vi "GVSGet Window Temp Reference.vi"(8 "sWindowName":string, 9 "sVIFullName":path, 10 "pVIRef_In":refnum<vi>, 11 "sAction":string) -> (0 "bResult":bool=TRUE, 1 "nWinType":i32, 2 "sTitleName Out":string, 3 "pVIRef_Out":refnum<vi>, 4 "sIcon_Out":string)   [LabVIEW 2013]
uses:
  <vilib>/Utility/miscctls.llb/LVPointTypeDef.ctl
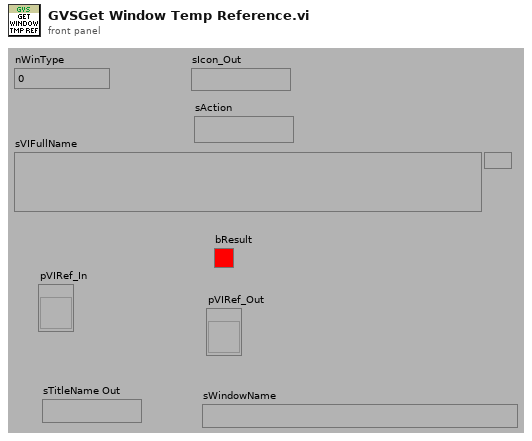
[diagram p1: front panel]
types:
  T1 = enum32{"Invalid", "Default", "Floating", "Floating/Auto-Hide", "Modal"}
  T2 = enum32{"Invalid", "Standard", "Closed", "Hidden", "Minimized", "Maximized"}
  T3 = typedef "LVPointTypeDef.ctl" = cluster{"Horizontal":i16, "Vertical":i16}
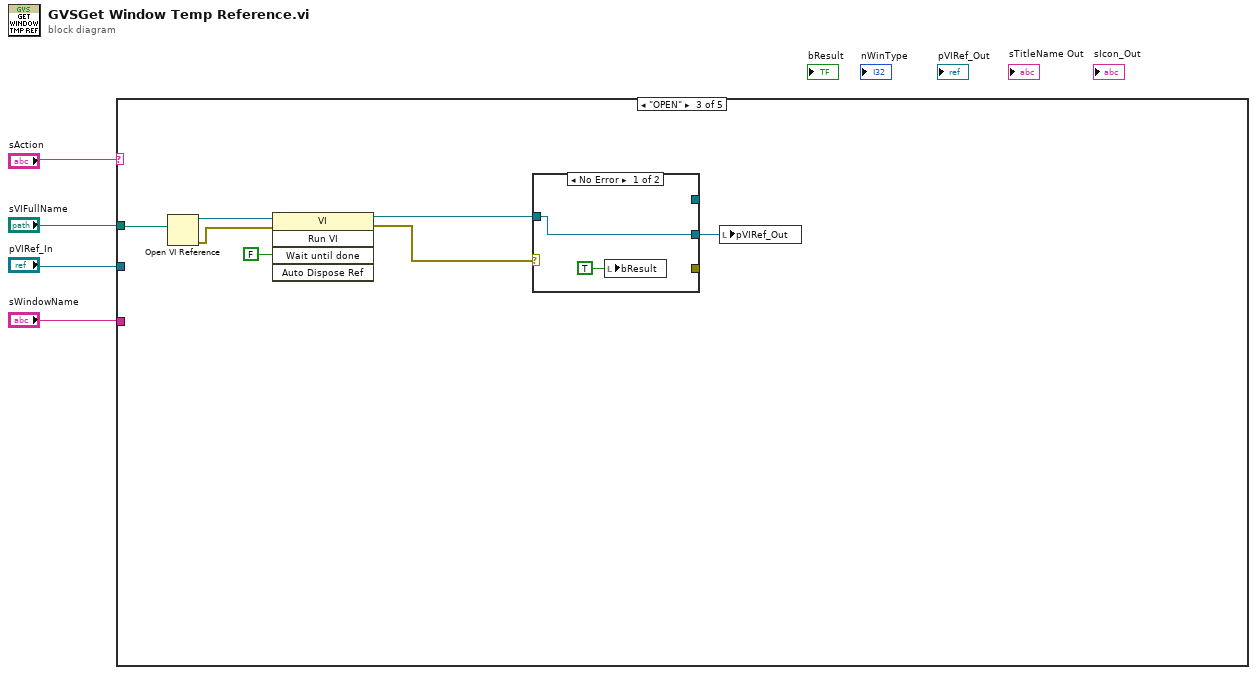
[diagram p0: block diagram]
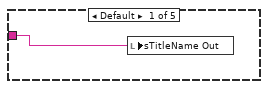
[diagram p2: hidden frame]
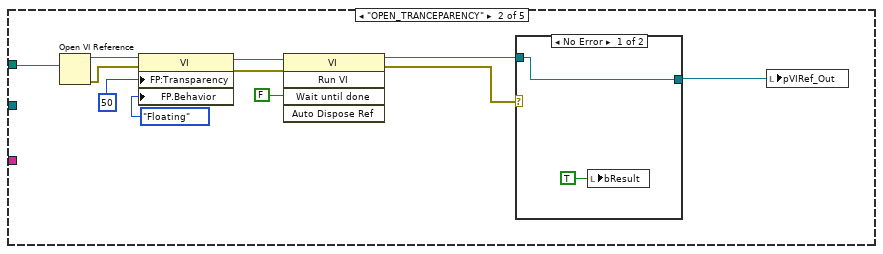
[diagram p3: hidden frame]
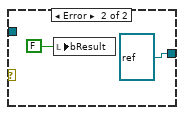
[diagram p4: hidden frame]
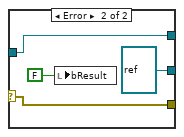
[diagram p5: hidden frame]
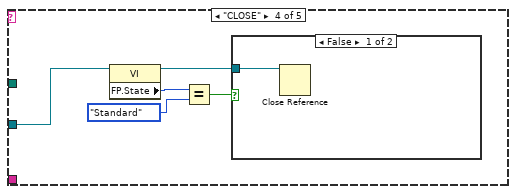
[diagram p6: hidden frame]
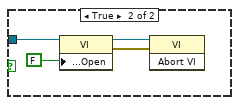
[diagram p7: hidden frame]
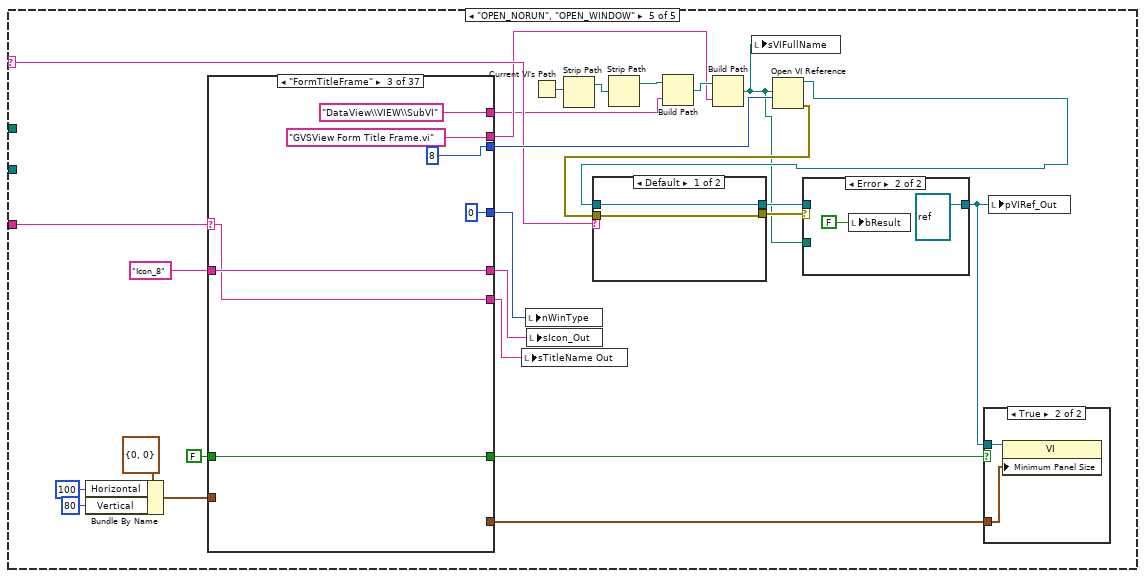
[diagram p8: hidden frame]
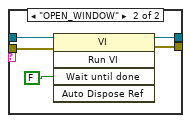
[diagram p10: hidden frame]
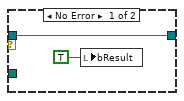
[diagram p11: hidden frame]
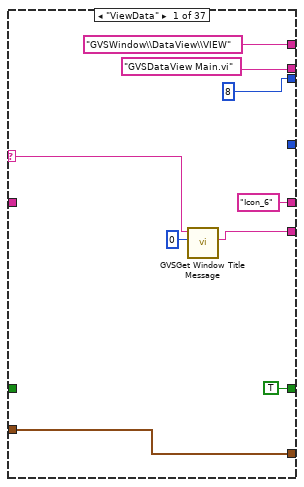
[diagram p12: hidden frame]
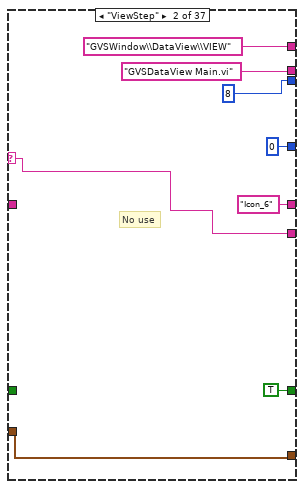
[diagram p13: hidden frame]
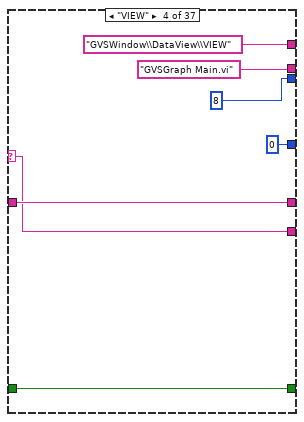
[diagram p14: hidden frame]
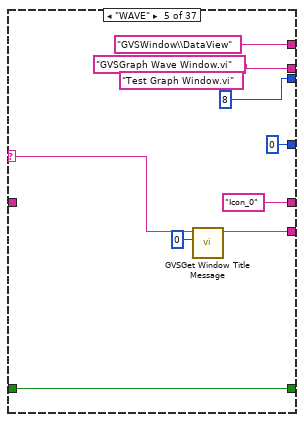
[diagram p15: hidden frame]
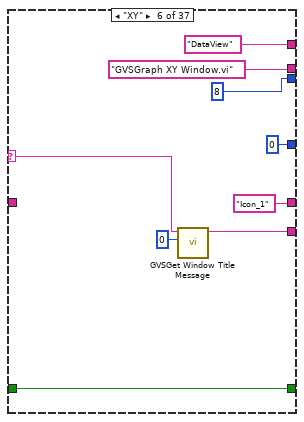
[diagram p16: hidden frame]
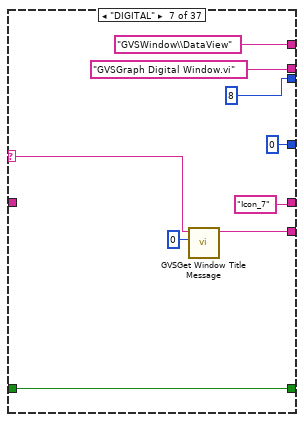
[diagram p17: hidden frame]
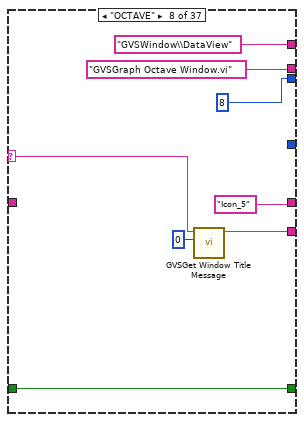
[diagram p18: hidden frame]
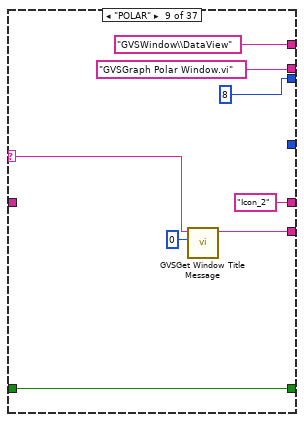
[diagram p19: hidden frame]
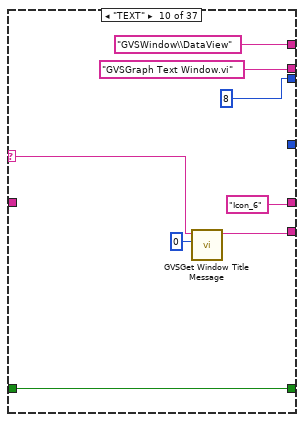
[diagram p20: hidden frame]
diagram:
  n1 = case shown="\"OPEN\"" "sAction" {
    selector: "sAction" -> [_ _ _ _ w61]
    tunnel: "sVIFullName" -> [_ w7 w24 _ _]
    tunnel: "pVIRef_In" -> [_ _ _ w36 _]
    tunnel: "sWindowName" -> [w5 _ _ _ w48]
    frame Default {
      n2 = local write "sTitleName Out"(w5) -> ()
    }
    frame "OPEN_TRANCEPARENCY" {
      n3 = Open VI Reference(vi path=w7) -> (vi reference=w12:refnum<vi>, error out=w13:errorcluster)  [unwired: 1 in, 4 out]
      n4 = property class="VI"(reference=w12, error in=w13, "FP:Transparency"=u8 50 ("Front Panel Window:Transparency"), "FP.Behavior"=T1."Floating" ("Front Panel Window:Behavior")) -> (reference out=w15:refnum<vi>, error out=w16:errorcluster)
      n5 = invoke class="VI" method="Run VI"(reference=w15, error in=w16, "Wait until done"=FALSE ("Wait Until Done")) -> (reference out=w8:refnum<vi>, error out=w9:errorcluster)  [unwired: 2 in, 3 out]
      n6 = case shown="No Error" w9 {
        tunnel: w8 -> [w17 _]
        tunnel: [w17 refnum<vi> refnum ("VIRef")] -> w6
        frame No Error {
          n7 = local write "bResult"(TRUE ("bResult")) -> ()
        }
        frame Error {
          n8 = local write "bResult"(FALSE ("bResult")) -> ()
        }
      }
      n9 = local write "pVIRef_Out"(w6) -> ()
    }
    frame "OPEN" {
      n10 = Open VI Reference(vi path=w24) -> (vi reference=w23:refnum<vi>, error out=w22:errorcluster)  [unwired: 1 in, 4 out]
      n11 = invoke class="VI" method="Run VI"(reference=w23, error in=w22, "Wait until done"=FALSE ("Wait Until Done")) -> (reference out=w25:refnum<vi>, error out=w26:errorcluster)  [unwired: 2 in, 3 out]
      n12 = case shown="No Error" w26 {
        selector: w26 -> [_ w30]
        tunnel: w25 -> [w28 w31]
        tunnel: [w28 refnum<vi> refnum ("VIRef_Out")] -> w21
        tunnel: [_ w31] -> _
        tunnel: [_ w30] -> _
        frame No Error {
          n13 = local write "bResult"(TRUE ("bResult")) -> ()
        }
        frame Error {
          n14 = local write "bResult"(FALSE ("bResult")) -> ()
        }
      }
      n15 = local write "pVIRef_Out"(w21) -> ()
    }
    frame "CLOSE" {
      n16 = property class="VI"(reference=w36) -> (reference out=w34:refnum<vi>, "FP.State"=w38:T2)  [unwired: 1 in, 1 out]
      n17 = Equal?(x=w38, y=T2."Standard" ("Front Panel Window:State")) -> (x = y?=w35:bool)
      n18 = case shown="False" w35 {
        tunnel: w34 -> [w39 w42]
        frame False {
          n19 = Close Reference(reference=w39) -> ()  [unwired: 1 in, 1 out]
        }
        frame True {
          n20 = property class="VI"(reference=w42, "Front Panel.Open"=FALSE ("Front Panel Window:Open")) -> (reference out=w41:refnum<vi>, error out=w40:errorcluster)  [unwired: 1 in]
          n21 = invoke class="VI" method="Abort VI"(reference=w41, error in=w40) -> ()  [unwired: 1 in, 3 out]
        }
      }
    }
    frame "OPEN_NORUN", "OPEN_WINDOW" {
      n22 = Bundle By Name(cluster=T3 {"Horizontal"=0, "Vertical"=0} ("Front Panel Window:Minimum Size"), "Horizontal"=i16 100, "Vertical"=i16 80) -> (w51:T3)
      n23 = case shown="\"FormTitleFrame\"" w48 {
        selector: w48 -> [w87 w95 w102 w110 w117 w126 w135 w143 w151 w159 w167 w175 w183 w191 w200 w207 w218 w226 w235 w242 w248 w254 w260 w268 w275 w281 w287 w293 w299 w307 w314 w320 w327 w333 w339 w345 w351]
        tunnel: ["GVSWindow\\DataView\\VIEW" ("name") "GVSWindow\\DataView\\VIEW" ("name") "DataView\\VIEW\\SubVI" ("name") "GVSWindow\\DataView\\VIEW" ("name") "GVSWindow\\DataView" ("name") "DataView" ("name") "GVSWindow\\DataView" ("name") "GVSWindow\\DataView" ("name") "GVSWindow\\DataView" ("name") "GVSWindow\\DataView" ("name") "GVSWindow\\DataView" ("name") "GVSWindow\\DataView" ("name") "GVSWindow\\DataView" ("name") "GVSWindow\\DataView" ("name") "GVSStepSetup" ("name") "GVSStepSetup" ("name") "GVSDocument" ("name") "GVSDocument" ("name") "GVSCurveLibrary" ("name") "GVSCurveLibrary\\SubVI" ("name") "GVSCurveLibrary\\SubVI" ("name") "GVSCurveLibrary\\SubVI" ("name") "GVSCurveLibrary\\SubVI" ("name") "GVSProject" ("name") "GVSSystem\\Misc" ("name") "GVSSystem\\Misc" ("name") "GVSSystem\\Misc" ("name") "GVSSystem\\Misc" ("name") "GVSWindow\\SubVI" ("name") "GVSAddStep" ("name") "GVSWindow\\SubVI" ("name") "GVSWindow\\SubVI" ("name") "GVSWindow\\SubVI" ("name") "GVSWindow\\SubVI" ("name") "GVSWindow\\SubVI" ("name") "GVSSystem\\Misc" ("name") "GVSWindow\\SubVI" ("name")] -> w50
        tunnel: ["GVSDataView Main.vi" ("name") "GVSDataView Main.vi" ("name") "GVSView Form Title Frame.vi" ("name") "GVSGraph Main.vi" ("name") "GVSGraph Wave Window.vi" ("name") "GVSGraph XY Window.vi" ("name") "GVSGraph Digital Window.vi" ("name") "GVSGraph Octave Window.vi" ("name") "GVSGraph Polar Window.vi" ("name") "GVSGraph Text Window.vi" ("name") "GVSGraph Table Window.vi" ("name") "GVSGraph Picture Window.vi" ("name") "GVSGraph Result Window.vi" ("name") "GVSGraph Intensity Window.vi" ("name") "GVSStepSetup.vi" ("name") "GVSStep Setup Default Window.vi" ("name") "GVSReport Main.vi" ("name") "SubVI\\GVSReport Frame.vi" ("name") "GVSCurve Library.vi" ("name") "GVSProbe Curve.vi" ("name") "GVSProbe Value.vi" ("name") "GVSProbe Result.vi" ("name") "GVSProbe Waveform.vi" ("name") "GVSProject Editor.vi" ("name") "GVSSignal Generator.vi" ("name") "GVSMultimeter.vi" ("name") "GVSScope-FFT.vi" ("name") "GVSRTA.vi" ("name") "GVSAPI TAB MAIN.vi" ("name") "GVSAdd Steps.vi" ("name") "GVSAPI Splitter Vertical.vi" ("name") "GVSAPI Splitter Horizontal.vi" ("name") "GVSAPI Temp Empty.vi" ("name") "GVSAPI Temp Frame.vi" ("name") "GVSAPI MSG PRO.vi" ("name") "GVSOperator Message.vi" ("name") "GVSAPI Temp Default.vi" ("name")] -> w59
        tunnel: [_ 0 0 0 0 0 0 _ _ _ _ _ _ _ _ _ _ _ _ _ _ _ _ _ _ _ _ _ _ _ _ 0 _ _ _ _ _] -> w65
        tunnel: "Icon_8" ("sIcon_Out") -> [_ _ w104 w112 _ _ _ _ _ _ _ _ _ _ _ w210 _ _ w230 w244 w249 w255 w261 _ _ _ _ _ w301 _ w316 w322 w329 w335 w341 w347 w353]
        tunnel: ["Icon_6" ("sIcon_Out") "Icon_6" ("sIcon_Out") w104 w112 "Icon_0" ("sIcon_Out") "Icon_1" ("sIcon_Out") "Icon_7" ("sIcon_Out") "Icon_5" ("sIcon_Out") "Icon_2" ("sIcon_Out") "Icon_6" ("sIcon_Out") "Icon_3" ("sIcon_Out") "Icon_8" ("sIcon_Out") "Icon_4" ("sIcon_Out") "Icon_9" ("sIcon_Out") "Icon_3" ("sIcon_Out") w210 "Icon_4" ("sIcon_Out") "Icon_6" ("sIcon_Out") w230 w244 w249 w255 w261 "Icon_1" ("sIcon_Out") "Icon_8" ("sIcon_Out") "Icon_8" ("sIcon_Out") "Icon_8" ("sIcon_Out") "Icon_8" ("sIcon_Out") w301 "Icon_7" ("sIcon_Out") w316 w322 w329 w335 w341 w347 w353] -> w63
        tunnel: [8 ("options") 8 ("options") 8 ("options") 8 ("options") 8 ("options") 8 ("options") 8 ("options") 8 ("options") 8 ("options") 8 ("options") 8 ("options") 8 ("options") 8 ("options") 8 ("options") 8 ("options") 8 ("options") 8 ("options") 8 ("options") 0 ("options") 8 ("options") 8 ("options") 8 ("options") 8 ("options") 0 ("options") 8 ("options") 8 ("options") 8 ("options") 8 ("options") 8 ("options") 0 ("options") 8 ("options") 8 ("options") 8 ("options") 8 ("options") 8 ("options") 0 ("options") 8 ("options")] -> w62
        tunnel: [w86 w95 w102 w110 w115 w124 w133 w141 w149 w157 w165 w173 w181 w189 w199 w207 w217 w226 w234 w242 w248 w254 w260 w267 w275 w281 w287 w293 w299 w306 w314 w320 w327 w333 w339 w345 w351] -> w60
        tunnel: FALSE -> [_ _ w101 w109 w116 w125 w134 w142 w150 w158 w166 w174 w182 w190 _ w206 _ w224 _ w241 w247 w253 w259 _ w274 w280 w286 w292 w298 _ w313 w319 w326 w332 w338 w344 w350]
        tunnel: [TRUE TRUE w101 w109 w116 w125 w134 w142 w150 w158 w166 w174 w182 w190 TRUE w206 TRUE w224 TRUE w241 w247 w253 w259 TRUE w274 w280 w286 w292 w298 TRUE w313 w319 w326 w332 w338 w344 w350] -> w56
        tunnel: [w84 w93 _ _ _ _ _ _ _ _ _ _ _ _ w197 _ w213 _ w232 _ _ _ _ w265 _ _ _ _ _ w304 _ _ _ _ _ _ _] -> w55
        tunnel: w51 -> [w84 w93 _ _ _ _ _ _ _ _ _ _ _ _ w197 _ _ _ w232 _ _ _ _ w265 _ _ _ _ _ w304 _ _ _ _ _ _ _]
        frame "ViewData" {
          n24 = call "GVSGet Window Title Message.vi"("No"=0 ("Error No"), "Kind"=w87) -> ("Unicode String"=w86:string)  [unwired: 4 in, 5 out]
        }
        frame "ViewStep" {
          # "No use"
        }
        frame "FormTitleFrame" {
        }
        frame "VIEW" {
        }
        frame "WAVE" {
          (unwired) "Test Graph Window.vi" ("name")
          n25 = call "GVSGet Window Title Message.vi"("No"=0 ("Error No"), "Kind"=w117) -> ("Multibyte String"=w115:string)  [unwired: 4 in, 5 out]
        }
        frame "XY" {
          n26 = call "GVSGet Window Title Message.vi"("No"=0 ("Error No"), "Kind"=w126) -> ("Multibyte String"=w124:string)  [unwired: 4 in, 5 out]
        }
        frame "DIGITAL" {
          n27 = call "GVSGet Window Title Message.vi"("No"=0 ("Error No"), "Kind"=w135) -> ("Multibyte String"=w133:string)  [unwired: 4 in, 5 out]
        }
        frame "OCTAVE" {
          n28 = call "GVSGet Window Title Message.vi"("No"=0 ("Error No"), "Kind"=w143) -> ("Multibyte String"=w141:string)  [unwired: 4 in, 5 out]
        }
        frame "POLAR" {
          n29 = call "GVSGet Window Title Message.vi"("No"=0 ("Error No"), "Kind"=w151) -> ("Multibyte String"=w149:string)  [unwired: 4 in, 5 out]
        }
        frame "TEXT" {
          n30 = call "GVSGet Window Title Message.vi"("No"=0 ("Error No"), "Kind"=w159) -> ("Multibyte String"=w157:string)  [unwired: 4 in, 5 out]
        }
        frame "TABLE" {
          n31 = call "GVSGet Window Title Message.vi"("No"=0 ("Error No"), "Kind"=w167) -> ("Multibyte String"=w165:string)  [unwired: 4 in, 5 out]
        }
        frame "PICTURE" {
          n32 = call "GVSGet Window Title Message.vi"("No"=0 ("Error No"), "Kind"=w175) -> ("Multibyte String"=w173:string)  [unwired: 4 in, 5 out]
        }
        frame "RESULT" {
          n33 = call "GVSGet Window Title Message.vi"("No"=0 ("Error No"), "Kind"=w183) -> ("Multibyte String"=w181:string)  [unwired: 4 in, 5 out]
        }
        frame "INTENSITY" {
          n34 = call "GVSGet Window Title Message.vi"("No"=0 ("Error No"), "Kind"=w191) -> ("Multibyte String"=w189:string)  [unwired: 4 in, 5 out]
        }
        frame "Step Setup" {
          n35 = call "GVSGet Window Title Message.vi"("No"=0 ("Error No"), "Kind"=w200) -> ("Unicode String"=w199:string)  [unwired: 4 in, 5 out]
        }
        frame "Step Setup Default" {
        }
        frame "Document" {
          n36 = Bundle By Name(cluster=T3 {"Horizontal"=0, "Vertical"=0} ("Front Panel Window:Minimum Size"), "Horizontal"=i16 300, "Vertical"=i16 200) -> (w213:T3)
          n37 = call "GVSGet Window Title Message.vi"("No"=0 ("Error No"), "Kind"=w218) -> ("Unicode String"=w217:string)  [unwired: 4 in, 5 out]
        }
        frame "ReportFrame" {
        }
        frame "Curves Library" {
          n38 = disable-structure shown="Disabled" {
            disable-tunnel: [w240 _] -> w231
            disable-tunnel: [w239 _] -> _
            frame Disabled {
              n39 = call "GVSGet Title Name and Icon from Type.vi"() -> ("Icon Name"=w239:string, "Title No"=w240:i32)  [unwired: 10 in]
            }
            frame Enabled {
            }
          }
          n40 = call "GVSGet Window Title Message.vi"("No"=w231, "Kind"=w235) -> ("Unicode String"=w234:string)  [unwired: 4 in, 5 out]
        }
        frame "Probe Curve" {
        }
        frame "Probe Value" {
        }
        frame "Probe Result" {
        }
        frame "Probe Waveform" {
        }
        frame "Project" {
          n41 = call "GVSGet Window Title Message.vi"("No"=0 ("Error No"), "Kind"=w268) -> ("Unicode String"=w267:string)  [unwired: 4 in, 5 out]
        }
        frame "Signal Generator" {
        }
        frame "Multimeter" {
        }
        frame "Oscilloscope-FFT" {
        }
        frame "RTA" {
        }
        frame "TAB" {
        }
        frame "Add Step" {
          n42 = call "GVSGet Window Title Message.vi"("No"=0 ("Error No"), "Kind"=w307) -> ("Unicode String"=w306:string)  [unwired: 4 in, 5 out]
        }
        frame "MainVertSplitter" {
        }
        frame "MainHorizSplitter" {
        }
        frame "CenterEmpty" {
        }
        frame "BasicWindow" {
        }
        frame "MsgProcesser" {
        }
        frame "Operator Msg Proc" {
        }
        frame Default {
        }
      }
      n43 = local write "sTitleName Out"(w60) -> ()
      n44 = local write "nWinType"(w65) -> ()
      n45 = local write "sIcon_Out"(w63) -> ()
      n46 = Current VI's Path() -> (path=w47:path)
      n47 = Strip Path(path=w47) -> (stripped path=w46:path)  [unwired: 1 out]
      n48 = Strip Path(path=w46) -> (stripped path=w44:path)  [unwired: 1 out]
      n49 = Build Path(base path=w44, name or relative path=w50) -> (appended path=w69:path)
      n50 = Build Path(base path=w69, name or relative path=w59) -> (appended path=w45:path)
      n51 = local write "sVIFullName"(w45) -> ()
      n52 = Open VI Reference(vi path=w45, options=w62) -> (vi reference=w49:refnum<vi>, error out=w67:errorcluster)  [unwired: 1 in, 3 out]
      n53 = case shown="Default" w61 {
        tunnel: [w72 w77] -> w68
        tunnel: w49 -> [w73 w76]
        tunnel: w67 -> [w72 w75]
        tunnel: [w73 w74] -> w66
        frame Default {
        }
        frame "OPEN_WINDOW" {
          n54 = invoke class="VI" method="Run VI"(reference=w76, error in=w75, "Wait until done"=FALSE ("Wait Until Done")) -> (reference out=w74:refnum<vi>, error out=w77:errorcluster)  [unwired: 2 in, 3 out]
        }
      }
      n55 = case shown="Error" w68 {
        tunnel: [w79 refnum<vi> refnum ("VIRef_Out")] -> w58
        tunnel: w66 -> [w79 _]
        tunnel: w45 -> [_ _]
        frame No Error {
          n56 = local write "bResult"(TRUE ("bResult")) -> ()
        }
        frame Error {
          n57 = local write "bResult"(FALSE ("bResult")) -> ()
        }
      }
      n58 = case shown="True" w56 {
        tunnel: w58 -> [_ w71]
        tunnel: w55 -> [_ w70]
        frame False {
        }
        frame True {
          n59 = property class="VI"(reference=w71, "Minimum Panel Size"=w70) -> ()  [unwired: 1 in, 2 out]
        }
      }
      n60 = local write "pVIRef_Out"(w58) -> ()
    }
  }
